vi "Win_PowerAmplifier_Transmit.vi"(8 "error in":errorcluster caption="错误输入") -> (0 "error out":errorcluster caption="错误输出", 1 "Yes out":bool=TRUE)   [LabVIEW 2020]
uses:
  <vilib>/Utility/xml.llb/Write to XML File(string).vi
panel:
  in  "Transmit":string[][](table)=[["33C", "0", "8", "02", "00", "00", "00", "00", "00", "00", "00", "100"], ["35C", "0", "8", "14", "00", "A9", "80", "4A", "94", "A0", "09", "100"], ["395", "0", "8", "00", "00", "00", "00", "00", "00", "00", "00", "100"], ["581", "0", "8", "81", "00", "00", "00", "00", "00", "00", "00", "500"], ["38F", "0", "8", "00", "00", "00", "00", "00", "00", "00", "00", "100"], ["", "", "", "", "", "", "", "", "", "", "", ""]]
  in  "No":bool
  in  "Yes":bool
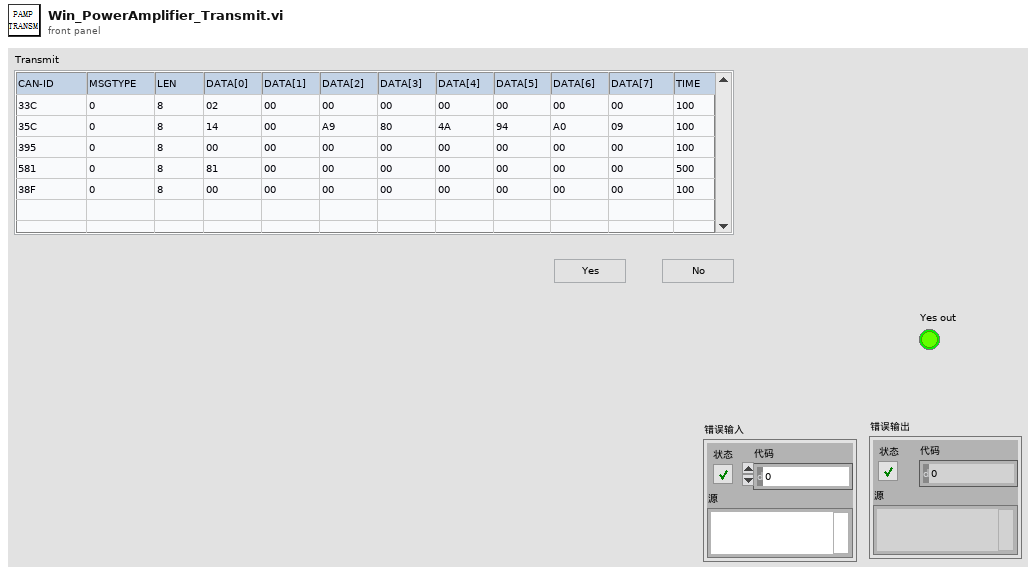
[diagram p1: front panel]
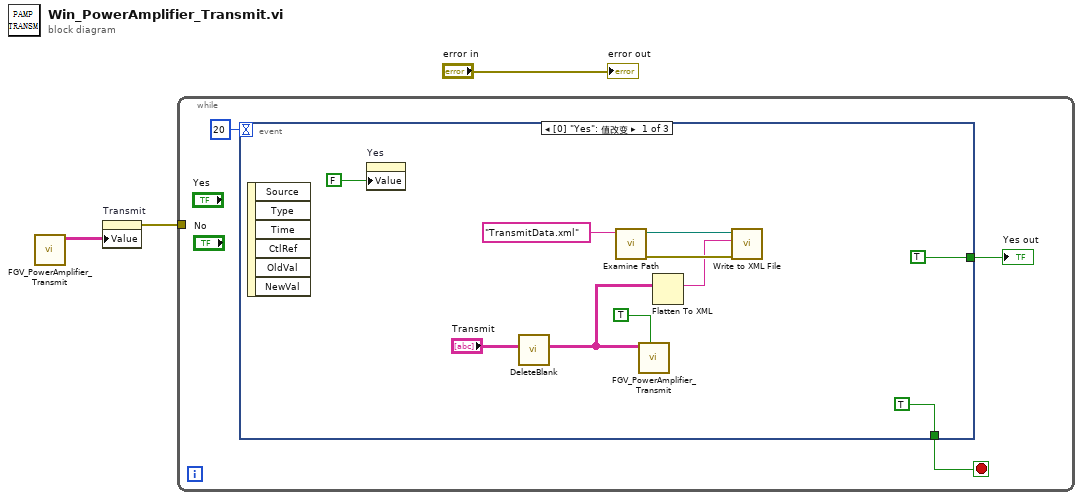
[diagram p0: block diagram]
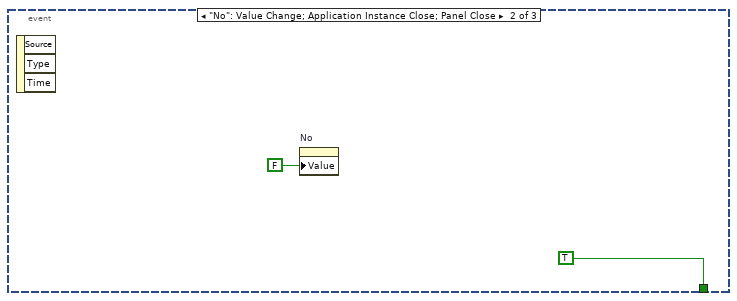
[diagram p2: hidden frame]
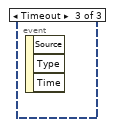
[diagram p3: hidden frame]
diagram:
  n1 = call "FGV_PowerAmplifier_Transmit.vi"() -> ("Transmit out"=w1:string[][])  [unwired: 10 in, 1 out]
  n2 = property on="Transmit" class="Tbl (严格)"("Value"=w1) -> (error out=w2:errorcluster)  [unwired: 2 in, 1 out]
  n3 = while {
    tunnel: w2 -> [_]
    stop <- w5 stop-if-true
    n4 = event shown="[0] \"Yes\": 值改变" {
      selector: _ -> [_ _ _]
      dyn-events: _ -> [_ _ _]
      timeout: 20 -> [_ _ _]
      tunnel: [TRUE TRUE _] -> w5
      tunnel: [TRUE _ _] -> w4
      event "Yes": Value Change {
        n5 = event-data() -> ()  [unwired: 1 in, 6 out]
        n6 = property on="Yes" class="Bool (严格)"("Value"=FALSE ("Yes")) -> ()  [unwired: 2 in, 2 out]
        n7 = call "DeleteBlank.vi"("Transmit"="Transmit") -> ("Transmit out"=w7:string[][])  [unwired: 10 in]
        n8 = call "Examine Path.vi"("Filename"="TransmitData.xml") -> ("error out"=w10:errorcluster, "Path"=w11:path)  [unwired: 9 in]
        n9 = call "FGV_PowerAmplifier_Transmit.vi"("Write?"=TRUE, "Transmit"=w7) -> ()  [unwired: 8 in, 2 out]
        n10 = Flatten To XML(6:w7) -> (2:w9:string)
        n11 = call-poly <vilib>:"Write to XML File.vi"("error in (no error)"=w10, "XML Input"=w9, "XML File Path"=w11) -> ()  [unwired: 6 in, 3 out]
      }
      event "No": Value Change; Application Instance Close; Panel Close {
        n12 = event-data() -> ()  [unwired: 1 in, 3 out]
        n13 = property on="No" class="Bool (严格)"("Value"=FALSE ("No")) -> ()  [unwired: 2 in, 2 out]
      }
      event Timeout {
        n14 = event-data() -> ()  [unwired: 1 in, 3 out]
      }
    }
    "Yes out" <- w4
  }
  "error out" <- "error in"
